vi "Convert_DC_VoltPct.vi"(1 "DC_Volt":dbl[unit]) -> (0 "DC_Volt%":dbl)   [LabVIEW 2024]
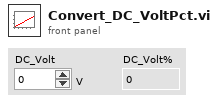
[diagram p1: front panel]
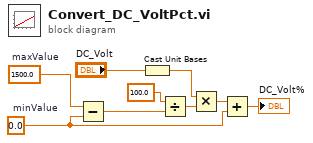
[diagram p0: block diagram]
diagram:
  w8 = 1500.0  # maxValue
  w5 = 0.0  # minValue
  n1 = Subtract(x=w8, y=w5) -> (x-y=w7:dbl)
  n2 = Cast Unit Bases(0:"DC_Volt") -> (2:w3:dbl)  [unwired: 1 in]
  n3 = Divide(x=100.0 ("y"), y=w7) -> (x/y=w6:dbl)
  n4 = Multiply(x=w3, y=w6) -> (x*y=w9:dbl)
  n5 = Add(x=w9, y=w5) -> (x+y=→"DC_Volt%":dbl)
